vi "Stop Acquisition.vi"(8 "error in (no error)":errorcluster, 11 "TroSpec in":refnum<class "PL ISTEQ TroSpec.lvclass">) -> (0 "error out":errorcluster, 3 "TroSpec out":refnum<class "PL ISTEQ TroSpec.lvclass">)   [LabVIEW 2015, in "PL ISTEQ TroSpec.lvclass"]
doc: "Stops frame acquisition."
uses:
  PL ISTEQ TroSpec.lvclass
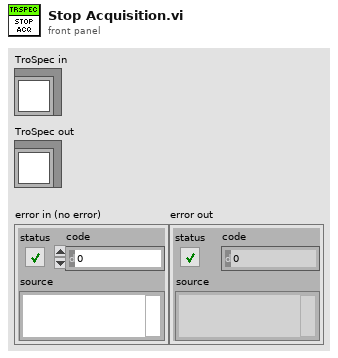
[diagram p1: front panel]
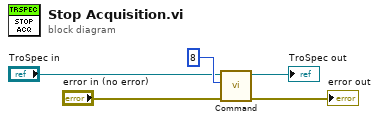
[diagram p0: block diagram]
diagram:
  n1 = call "Command.vi"("error in (no error)"="error in (no error)", "command"=u16 8 ("address"), "TroSpec in"="TroSpec in") -> ("error out"=→"error out":errorcluster, "TroSpec out"=→"TroSpec out":refnum<class "PL ISTEQ TroSpec.lvclass">)  [unwired: 6 in, 1 out]
